vi "Determine Sector Edge Location.vi"(11 "Preanalysis Stage":bool) -> (2 "Left Sector Edge":u8, 3 "Right Sector Edge":u8)   [LabVIEW 2013]
doc: "Takes the average sector intensities and compares each average to the threshold value to determine which sector the edge is located in."
uses:
  Globals/Accumulated Sector Intensity.vi
  Globals/Sector Parameter Global.vi
  <vilib>/rvi/FIFO/Fifo_Resource/nirvififoEmulationReadFpgaImpl.vi
  <vilib>/rvi/DataTransferAndStorage/Container/Common/niFpgaContainerGetUniqueNameForEmu.vi
  <vilib>/rvi/interface/RandomDataEmulation/nirviRandomDataFPGAFIFO.vi
  <vilib>/rvi/interface/RandomDataEmulation/niFpgaRandomDataHandleErrors.vi
  <vilib>/rvi/DataTransferAndStorage/Container/XNode/niFpgaContainer.xnode
  <vilib>/rvi/FIFO/Fifo_Resource/nirvififoEmulationRead.vi
  <vilib>/rvi/interface/RandomDataEmulation/nirviRandomDataFpgaReadWriteTemplate.vi
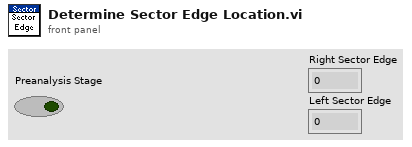
[diagram p1: front panel]
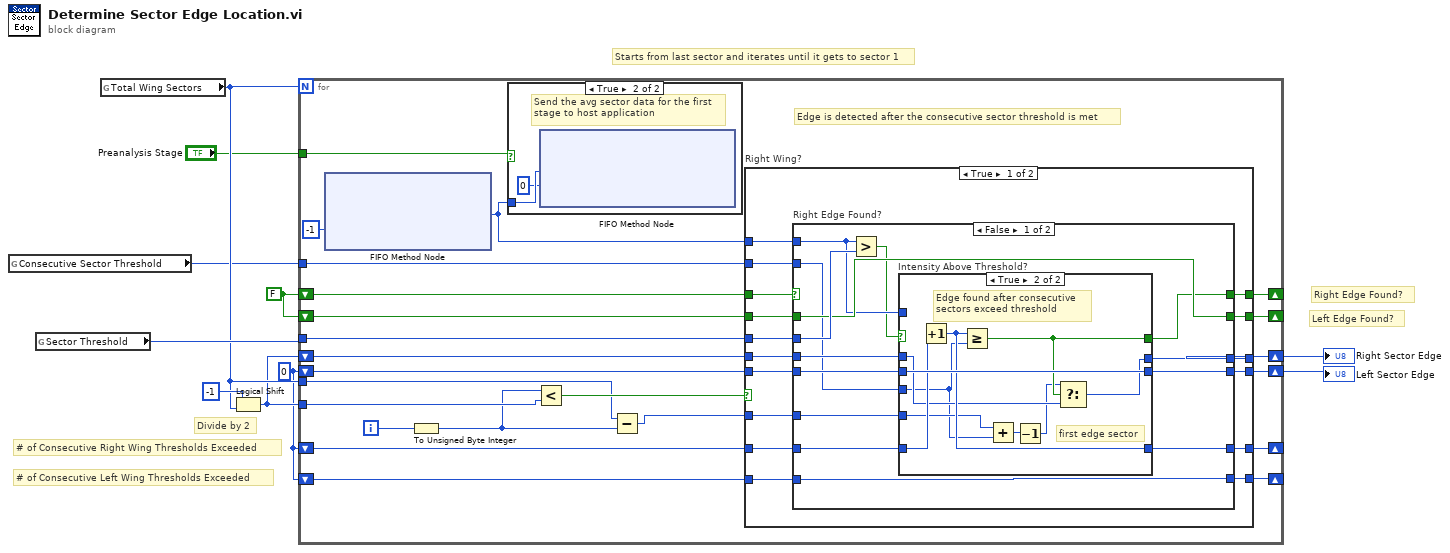
[diagram p0: block diagram]
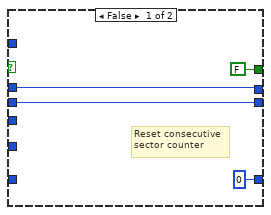
[diagram p3: hidden frame]
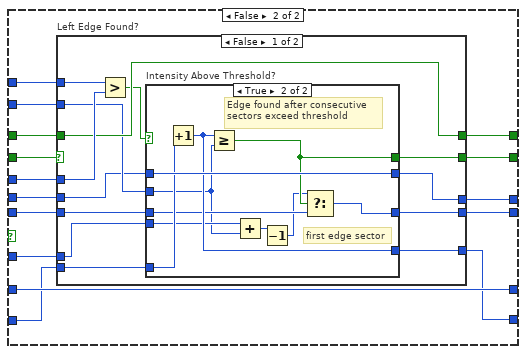
[diagram p5: hidden frame]
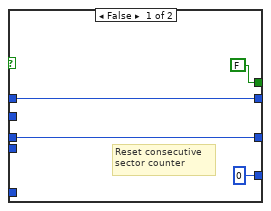
[diagram p6: hidden frame]
diagram:
  w2 = u8 0 ("Total Wing Sectors")
  w7 = FALSE ("Left Edge Found?")
  # "# of Consecutive Left Wing Thresholds Exceeded"
  # "# of Consecutive Right Wing Thresholds Exceeded"
  # "Starts from last sector and iterates until it gets to sector 1"
  # "Left Edge Found?"
  # "Right Edge Found?"
  # "Divide by 2"
  n1 = global read "Sector Parameter Global.vi" "Consecutive Sector Threshold"() -> (w1:u8)
  n2 = global read "Sector Parameter Global.vi" "Sector Threshold"() -> (w6:u8)
  n3 = global read "Accumulated Sector Intensity.vi" "Total Wing Sectors"() -> (w5:u8)
  n4 = Logical Shift(y=i16 -1, x=w5) -> (x << y=w3:u8)
  n5 = for {
    N: w5 -> [_]
    tunnel: w6 -> [w31]
    tunnel: w3 -> [w32]
    shift-right: [w29] -> _
    shift-left: w7 -> [w30]
    shift-right: [w22] -> _
    shift-left: w7 -> [w23]
    shift-right: [w27] -> w10
    shift-left: w3 -> [w26]
    shift-right: [w25] -> w9
    shift-left: w2 -> [w24]
    tunnel: w5 -> [w19]
    tunnel: "Preanalysis Stage" -> [w16]
    shift-right: [w13] -> _
    shift-left: w2 -> [w15]
    shift-right: [w12] -> _
    shift-left: w2 -> [w11]
    tunnel: w1 -> [w14]
    i -> [w28]
    # "Edge is detected after the consecutive sector threshold is met"
    n6 = xnode ("FIFO Method Node")("Timeout"=-1) -> ("Element"=w21:u8)  [unwired: 1 in, 2 out]
    n7 = To Unsigned Byte Integer(number=w28) -> (unsigned 8bit integer=w18:u8)
    n8 = case shown="True" w16 {
      tunnel: w21 -> [_ w35]
      frame False {
      }
      frame True {
        # "Send the avg sector data for the first\nstage to host application"
        n9 = xnode ("FIFO Method Node")("Element"=w35, "Timeout"=0) -> ()  [unwired: 1 in, 2 out]
      }
    }
    n10 = Less?(x=w18, y=w32) -> (x < y?=w33:bool)
    n11 = Subtract(x=w19, y=w18) -> (x-y=w17:u8)
    n12 = case "Right Wing?" shown="True" w33 {
      tunnel: w21 -> [w50 w100]
      tunnel: w31 -> [w49 w99]
      tunnel: w30 -> [w51 w91]
      tunnel: [w48 w98] -> w29
      tunnel: w17 -> [w47 w97]
      tunnel: [w46 w96] -> w27
      tunnel: w26 -> [w45 w95]
      tunnel: [w44 w94] -> w25
      tunnel: w24 -> [w43 w93]
      tunnel: w23 -> [w42 w92]
      tunnel: [w41 w90] -> w22
      tunnel: w15 -> [w40 w89]
      tunnel: w14 -> [w39 w86]
      tunnel: [w38 w89] -> w13
      tunnel: [w37 w87] -> w12
      tunnel: w11 -> [w36 w88]
      frame True {
        n13 = case "Right Edge Found?" shown="False" w51 {
          selector: w51 -> [_ w82]
          tunnel: w50 -> [w58 _]
          tunnel: w49 -> [w65 _]
          tunnel: [w54 w82] -> w48
          tunnel: w47 -> [w64 _]
          tunnel: [w63 w85] -> w46
          tunnel: w45 -> [w62 w85]
          tunnel: [w61 w84] -> w44
          tunnel: w43 -> [w60 w84]
          tunnel: w42 -> [w59 w83]
          tunnel: [w59 w83] -> w41
          tunnel: w40 -> [w57 w81]
          tunnel: w39 -> [w56 _]
          tunnel: [w53 w81] -> w38
          tunnel: [w52 w80] -> w37
          tunnel: w36 -> [w52 w80]
          frame False {
            n14 = Greater?(x=w58, y=w65) -> (0:w55:bool)
            n15 = case "Intensity Above Threshold?" shown="True" w55 {
              tunnel: w64 -> [_ w73]
              tunnel: [w69 w75] -> w63
              tunnel: w62 -> [w69 w74]
              tunnel: [w68 w79] -> w61
              tunnel: w60 -> [w68 w79]
              tunnel: w58 -> [_ _]
              tunnel: w57 -> [_ w78]
              tunnel: w56 -> [_ w72]
              tunnel: [FALSE w76] -> w54
              tunnel: [u8 0 w77] -> w53
              frame False {
                # "Reset consecutive\nsector counter"
              }
              frame True {
                # "first edge sector"
                # "Edge found after consecutive\nsectors exceed threshold"
                n16 = Increment(x=w78) -> (x+1=w77:u8)
                n17 = Greater Or Equal?(x=w77, y=w72) -> (x >= y?=w76:bool)
                n18 = Add(x=w73, y=w72) -> (x+y=w71:u8)
                n19 = Decrement(x=w71) -> (x-1=w70:u8)
                n20 = Select(t=w70, s=w76, f=w74) -> (s? t:f=w75:u8)
              }
            }
          }
          frame True {
          }
        }
      }
      frame False {
        n21 = case "Left Edge Found?" shown="False" w92 {
          selector: w92 -> [_ w129]
          tunnel: w100 -> [w111 _]
          tunnel: w99 -> [w113 _]
          tunnel: [w112 w130] -> w98
          tunnel: w97 -> [w104 _]
          tunnel: [w101 w132] -> w96
          tunnel: w95 -> [w102 w132]
          tunnel: [w106 w131] -> w94
          tunnel: w93 -> [w105 w131]
          tunnel: w91 -> [w112 w130]
          tunnel: [w108 w129] -> w90
          tunnel: w88 -> [w109 w128]
          tunnel: [w107 w128] -> w87
          tunnel: w86 -> [w103 _]
          frame False {
            n22 = Greater?(x=w111, y=w113) -> (0:w110:bool)
            n23 = case "Intensity Above Threshold?" shown="True" w110 {
              tunnel: w104 -> [_ w121]
              tunnel: [w117 w123] -> w106
              tunnel: w105 -> [w117 w122]
              tunnel: [w116 w127] -> w101
              tunnel: w102 -> [w116 w127]
              tunnel: w109 -> [_ w126]
              tunnel: w103 -> [_ w120]
              tunnel: [FALSE w124] -> w108
              tunnel: [u8 0 w125] -> w107
              frame False {
                # "Reset consecutive\nsector counter"
              }
              frame True {
                # "first edge sector"
                # "Edge found after consecutive\nsectors exceed threshold"
                n24 = Increment(x=w126) -> (x+1=w125:u8)
                n25 = Greater Or Equal?(x=w125, y=w120) -> (x >= y?=w124:bool)
                n26 = Add(x=w121, y=w120) -> (x+y=w119:u8)
                n27 = Decrement(x=w119) -> (x-1=w118:u8)
                n28 = Select(t=w118, s=w124, f=w122) -> (s? t:f=w123:u8)
              }
            }
          }
          frame True {
          }
        }
      }
    }
  }
  "Right Sector Edge" <- w10
  "Left Sector Edge" <- w9
